vi "Make Markers String.vi"(5 "Label (optional)":T1, 6 "Icon URL (optional)":string, 7 "Size (optional)":T2, 8 "error in (no error)":errorcluster, 10 "Array of Locations":string[](array[string]), 11 "Color (optional)":u32(colorbox)) -> (0 "error out":errorcluster, 2 "Markers string":string)   [LabVIEW 2012]
uses:
  TypeDefs/Marker Sizes.ctl
  TypeDefs/Marker Labels.ctl
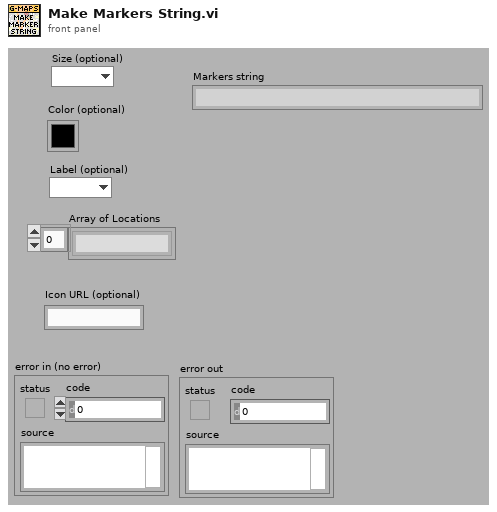
[diagram p1: front panel]
types:
  T1 = typedef "Marker Labels.ctl" = enum16{"", "A", "B", "C", "D", "E", "F", "G", "H", "I", "J", "K", "M", "N", "O", "P", "Q", "R", "S", "T", "U", "V", "W", "X", "Y", "Z", "1", "2", "3", "4", "5", "6", "7", "8", "9", "0"}
  T2 = typedef "Marker Sizes.ctl" = enum16{"", "small", "mid", "tiny"}
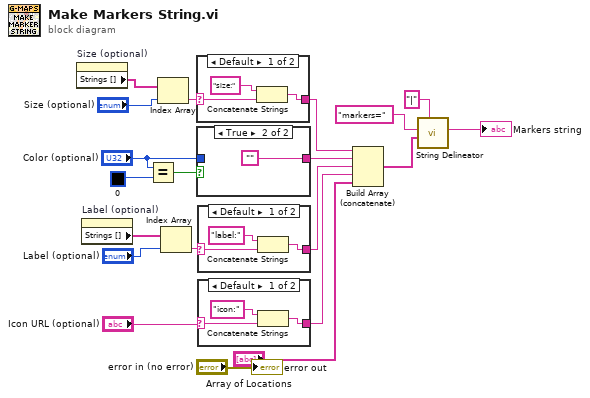
[diagram p0: block diagram]
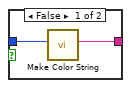
[diagram p3: hidden frame]
diagram:
  n1 = property on="Size (optional)" class="Enum (strict)"() -> ("Strings []"=w20:string[])  [unwired: 2 in, 2 out]
  n2 = property on="Label (optional)" class="Enum (strict)"() -> ("Strings []"=w18:string[])  [unwired: 2 in, 2 out]
  n3 = Equal?(x="Color (optional)", y=u32 0 ("Color (optional) 2")) -> (x = y?=w10:bool)
  n4 = Index Array(array=w20, index="Size (optional)") -> (element=w14:string)
  n5 = Index Array(array=w18, index="Label (optional)") -> (element=w13:string)
  n6 = case shown="Default" w14 {
    selector: w14 -> [w22 w24]
    tunnel: [w21 w24] -> w9
    frame Default {
      n7 = Concatenate Strings("size:" ("URL"), w22) -> (w21:string)
    }
    frame "" {
    }
  }
  n8 = case shown="True" w10 {
    tunnel: "Color (optional)" -> [w26 _]
    tunnel: [w25 ""] -> w8
    frame False {
      n9 = call "Make Color String.vi"("Color"=w26) -> ("color string"=w25:string)  [unwired: 9 in, 1 out]
    }
    frame True {
    }
  }
  n10 = case shown="Default" w13 {
    selector: w13 -> [w29 w31]
    tunnel: [w28 w31] -> w7
    frame Default {
      n11 = Concatenate Strings("label:" ("URL"), w29) -> (w28:string)
    }
    frame "" {
    }
  }
  n12 = case shown="Default" "Icon URL (optional)" {
    selector: "Icon URL (optional)" -> [w33 w35]
    tunnel: [w32 w35] -> w1
    frame Default {
      n13 = Concatenate Strings("icon:" ("URL"), w33) -> (w32:string)
    }
    frame "" {
    }
  }
  n14 = Build Array (concatenate)(w9, w8, w7, w1, "Array of Locations") -> (w6:string[])
  n15 = call "String Delineator.vi"("Delineator \"&\""="|" ("URL"), "Array of Strings"=w6, "Base String"="markers=" ("URL")) -> ("New String"=→"Markers string":string)  [unwired: 7 in, 1 out]
  "error out" <- "error in (no error)"
